vi "sub_distance_processing.vi"(0 "Magnitude high":dbl[](array[numeric]), 1 "Calibration":T2 {"r bias" format="%_3p"; "Ks" format="%#_3p"}, 3 "Measurements In":T1 {"RMS" format="%#_3p"; "Relative" format="%.4f"; "Ref distance" format="%.3f"; "DC" format="%.3f"}, 5 "Magnitude low":dbl, 9 "Modulation info":T3 {"Hi channels at low" min=0 step=1; "Low carriers" format="%#_6p"; "High carriers" format="%#_6p"}, 11 "Reset":bool, 12 "Output options":T4={"Source"=enum."X", "Sensor"=enum."X", "Sense"=FALSE, "Distance"=FALSE, "LF corner"=0.0, "RMS Tc"=5.0}, 13 "Reset RMS":bool, 14 "Time Stamp":timestamp) -> (4 "Measurements out":T1 {"RMS" format="%#_3p"; "Relative" format="%.4f"; "Ref distance" format="%.3f"; "DC" format="%.3f"}, 6 "Mean level":dbl[](array[numeric]), 10 "Chart display":waveform(dbl)[](array[waveform]), 15 "Distance high":dbl[](array[numeric]))   [LabVIEW 2026]
uses:
  gui/output_options.ctl
  gui/coupling_selector.ctl
  processing/modulation_info.ctl
  gui/measurements.ctl
  calibration.ctl
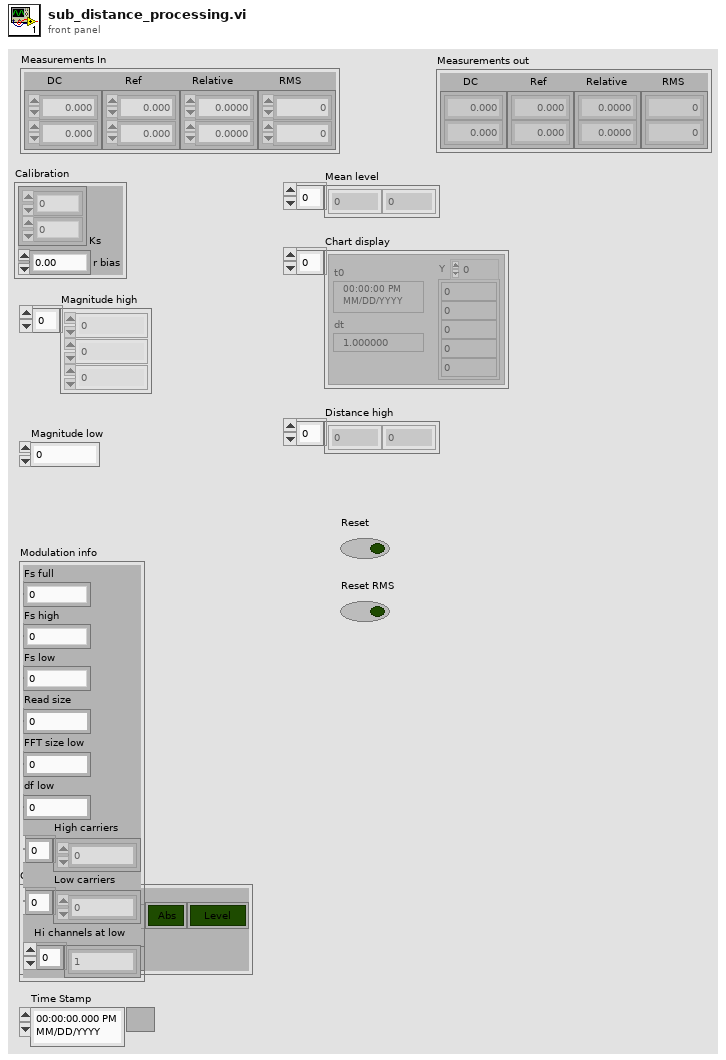
[diagram p1: front panel]
types:
  T1 = typedef "measurements.ctl" = cluster{"DC":dbl[], "Ref distance":dbl[], "Relative":dbl[], "RMS":dbl[]}
  T2 = typedef "calibration.ctl" = cluster{"Ks":dbl[], "r bias":dbl}
  T3 = typedef "modulation_info.ctl" = cluster{"Fs full":dbl, "Fs high":dbl, "Fs low":dbl, "Read size":i32, "FFT size low":i32, "df low":dbl, "High carriers":dbl[], "Low carriers":dbl[], "Hi channels at low":i32[]}
  T4 = typedef "output_options.ctl" = cluster{"Source":T5, "Sensor":T5, "Sense":bool, "Distance":bool, "LF corner":dbl, "RMS Tc":dbl}
  T5 = typedef "coupling_selector.ctl" = enum16{"X", "Y", "Z", "Vector"}
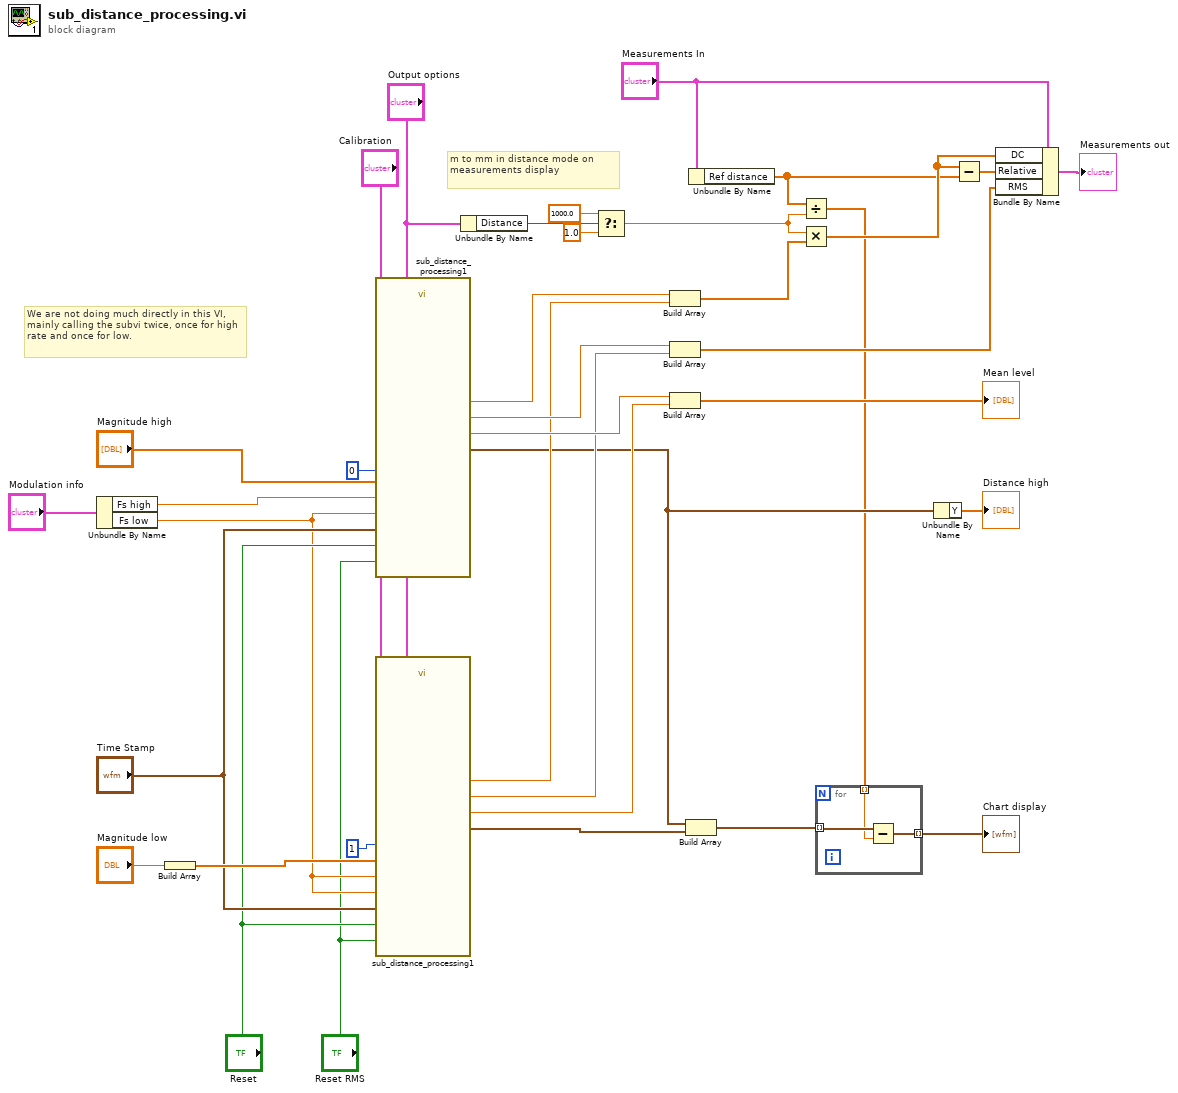
[diagram p0: block diagram]
diagram:
  # "We are not doing much directly in this VI, mainly calling the subvi twice, once for high rate and once for low."
  # "m to mm in distance mode on measurements display"
  n1 = Unbundle By Name("Modulation info") -> ("Fs high"=w21:dbl, "Fs low"=w15:dbl)
  n2 = Build Array("Magnitude low") -> (w18:dbl[])
  n3 = call "sub_distance_processing1.vi"("Calibration"="Calibration", "Reset RMS"="Reset RMS", "Output options"="Output options", "High/low index"=0, "Magnitude"="Magnitude high", "Fs low"=w15, "Fs"=w21, "Reset"="Reset", "Time Stamp"="Time Stamp") -> ("RMS"=w22:dbl, "DC"=w25:dbl, "Mean level"=w27:dbl, "Waveform"=w4:waveform(dbl))  [unwired: 3 in]
  n4 = call "sub_distance_processing1.vi"("Calibration"="Calibration", "Reset RMS"="Reset RMS", "Output options"="Output options", "High/low index"=1, "Magnitude"=w18, "Fs low"=w15, "Fs"=w15, "Reset"="Reset", "Time Stamp"="Time Stamp") -> ("RMS"=w11:dbl, "DC"=w12:dbl, "Mean level"=w10:dbl, "Waveform"=w9:waveform(dbl))  [unwired: 3 in]
  n5 = Unbundle By Name("Output options") -> ("Distance"=w37:bool)
  n6 = Select(t=1000.0, s=w37, f=1.0) -> (s? t:f=w3:dbl)
  n7 = Build Array(w25, w12) -> (w24:dbl[])
  n8 = Build Array(w22, w11) -> (w8:dbl[])
  n9 = Build Array(w27, w10) -> (→"Mean level":dbl[])
  n10 = Build Array(w4, w9) -> (w6:waveform(dbl)[])
  n11 = Unbundle By Name("Measurements In") -> ("Ref distance"=w2:dbl[])
  n12 = Divide(x=w2, y=w3) -> (x/y=w1:dbl[])
  n13 = Multiply(x=w3, y=w24) -> (x*y=w36:dbl[])
  n14 = for {
    tunnel: w6 -> [w40] mode=indexing
    tunnel: w1 -> [w39] mode=indexing
    tunnel: [w38] -> w5 mode=indexing
    n15 = Subtract(x=w40, y=w39) -> (x-y=w38:waveform(dbl))
  }
  "Chart display" <- w5
  n16 = Unbundle By Name(w4) -> ("Y"=→"Distance high":dbl[])
  n17 = Subtract(x=w36, y=w2) -> (x-y=w35:dbl[])
  n18 = Bundle By Name(cluster="Measurements In", "DC"=w36, "Relative"=w35, "RMS"=w8) -> (→"Measurements out":T1)
